vi "Part 2.vi"(11 "Input":string="on x=-44..5,y=-19..31,z=-15..33\non x=-39..11,y=-17..30,z=-15..30\non x=-42..10,y=-43..7,z=-4..40\non x=-4..47,y=-8..45,z=-8..43\non x=-18..28,y=-15..30,z=-36..12\non x=-24..24,y=-33..14,z=-49..1\non x=-14..30,y=-34..14,z=-27..24\non x=-45..7,y=-6..43,z=-9..41\non x=-16..37,y=-49..-5,z=-30..21\non x=-10..42,y=-35..10,z=-43..11\noff x=7..17,y=-8..5,z=-30..-18\non x=-49..3,y=-27..23,z=-44..1\noff x=10..23,y=-21..-10,z=-37..-19\non x=-41..4,y=-11..41,z=-36..16\noff x=-6..4,y=40..49,z=12..30\non x=-2..49,y=-43..3,z=-32..13\noff x=-44..-29,y=-8..6,z=1..17\non x=-9..36,y=-7..43,z=-37..14\noff x=-1..12,y=-36..-23,z=28..47\non x=-26..27,y=-45..3,z=-20..24\non x=-87853..-63955,y=-14079..10797,z=16618..34667\non x=-22600..-10441,y=-47268..-24491,z=-72641..-62383\non x=-7793..18488,y=71672..78114,z=-44666..-18458\non x=73..5701,y=-2494..28421,z=-89152..-65315\non x=-37051..-30202,y=15342..24015,z=-77231..-62996\non x=53246..70778,y=-62293..-47740,z=20277..41217\non x=-14142..12389,y=62146..65958,z=-55683..-41913\non x=-48728..-18398,y=8282..34289,z=-81114..-48336\non x=-59177..-22673,y=-49858..-29386,z=-59127..-47368\non x=-85434..-72245,y=13867..31427,z=-21594..-2631\non x=-35402..-12325,y=-37452..-19185,z=-81697..-63051\non x=61174..80227,y=-866..32461,z=-20053..-10077\non x=-32647..-1711,y=-35706..-20854,z=-72604..-60376\non x=59957..82200,y=-30164..2313,z=-30464..-19345\non x=6801..22281,y=24570..51370,z=-81154..-67264\non x=20369..39838,y=73729..88454,z=577..19763\non x=29800..52019,y=29499..61971,z=48435..55070\non x=28801..40411,y=-84420..-69983,z=-13267..2211\non x=13549..40576,y=-47493..-31658,z=-71685..-40487\non x=13137..24167,y=-66931..-49605,z=26517..54208\non x=33284..48135,y=46431..67202,z=48616..59067\non x=-56715..-26618,y=56864..79700,z=-25450..-654\non x=-54074..-25399,y=-52684..-36578,z=35631..52148\non x=37464..54023,y=-34067..-6521,z=-70559..-54490\non x=-41089..-11111,y=-47478..-29133,z=60940..74315\non x=-82774..-52991,y=-54204..-20897,z=23960..42825\non x=30749..49712,y=35786..69307,z=37491..45758\non x=-11491..14973,y=-93031..-58484,z=17353..44836\non x=-57064..-20188,y=-63440..-37103,z=47342..70176\non x=-27801..-375,y=30934..59690,z=45378..71236\non x=61123..82155,y=-15850..-525,z=-53874..-32638\non x=-16993..-2751,y=40182..64669,z=-62209..-45026\non x=-82058..-51602,y=6298..30885,z=-39693..-17573\non x=49260..58127,y=-59897..-48624,z=-30308..-16577\non x=-56788..-40095,y=-25293..-14542,z=-68269..-53982\non x=2505..5932,y=-47595..-22583,z=64838..84486\non x=-53828..-37906,y=-72105..-58994,z=-4913..17377\non x=5051..19306,y=77062..91570,z=-31347..-1735\non x=-16847..-320,y=-93124..-64459,z=12444..33910\non x=-45648..-18838,y=34175..55012,z=39079..55510\non x=63218..83253,y=-23970..-4735,z=2800..11596\non x=50244..76221,y=-50393..-33391,z=-17785..-7738\non x=35816..43139,y=-73177..-43183,z=-41697..-13098\non x=-66225..-48531,y=-36053..-16991,z=-48638..-26491\non x=-20786..8663,y=28061..38714,z=-84899..-63223\non x=59014..76501,y=10125..25324,z=-54183..-35850\non x=-24243..-8597,y=-47135..-12076,z=62724..76012\non x=-23347..7901,y=-81218..-55820,z=-60425..-30059\non x=56319..71652,y=23428..36372,z=-51760..-40670\non x=-13463..10312,y=78981..96298,z=-15494..17820\non x=25458..54307,y=-35736..-28250,z=48784..77696\non x=43259..63044,y=15682..26592,z=-71035..-52596\non x=-29348..-4953,y=54062..67679,z=39619..65019\non x=49369..63882,y=-39377..-21590,z=-53387..-47336\non x=13595..25896,y=27751..59875,z=-78381..-44266\non x=-62701..-44978,y=22333..30908,z=-54143..-42897\non x=7977..25840,y=-82123..-71218,z=-16092..-696\non x=72848..80580,y=-3963..7995,z=-14735..10441\non x=69499..92382,y=-2662..28065,z=-42992..-17994\non x=48475..68268,y=42740..64001,z=14503..39264\non x=-49063..-33385,y=-58610..-30409,z=41056..71840\non x=-59232..-33228,y=45184..76352,z=17766..31561\non x=5959..26638,y=-9552..20815,z=75305..87615\non x=47753..57971,y=42230..61946,z=-12647..-3804\non x=-81759..-73203,y=4440..38862,z=-16003..-3110\non x=-73980..-59456,y=-47097..-28017,z=-25117..7475\non x=23176..38914,y=50432..59832,z=31931..54668\non x=-71483..-48041,y=19572..30248,z=-40958..-32806\non x=-37783..-21743,y=-87276..-58240,z=-21390..-1919\non x=-18665..960,y=-5907..20986,z=66322..81301\non x=5286..37737,y=50107..67657,z=-67474..-42701\non x=31390..48914,y=-70366..-54470,z=-46904..-23117\non x=-27683..-15749,y=-47749..-34632,z=-76712..-50928\non x=-90781..-60103,y=-31150..-20145,z=-23382..5464\non x=-44373..-33411,y=55729..68596,z=-34550..-16532\non x=-1309..36490,y=-88067..-66282,z=-27329..-13890\non x=-70563..-54927,y=2742..28284,z=-59814..-41321\non x=36257..58977,y=52630..81787,z=-2016..28038\non x=59652..83384,y=-3386..9206,z=-40944..-13798\non x=-27792..6186,y=-47017..-27949,z=-75807..-45725\non x=60095..91023,y=-26573..-21046,z=-13267..10809\non x=-22369..-1689,y=-47418..-28289,z=-67790..-44667\non x=-73998..-62782,y=-24350..-3753,z=-44689..-24202\non x=-66355..-39116,y=26462..39518,z=44344..65908\non x=-82304..-51017,y=17614..36432,z=18664..50639\non x=-73956..-67827,y=18133..33852,z=-29108..-16920\non x=-79701..-67912,y=-30890..-20859,z=-11116..782\non x=60573..90823,y=-12009..12435,z=21040..48487\non x=-42470..-30925,y=18977..50582,z=-66812..-55290\non x=-44675..-19948,y=6997..36868,z=-76580..-55763\non x=-40167..-9959,y=-86179..-65330,z=22876..50418\non x=-14480..4184,y=-82281..-61373,z=-43344..-6589\non x=49703..56170,y=-12257..-3969,z=43782..66373\non x=37233..54010,y=-39264..-11480,z=-75787..-54270\non x=-63691..-41496,y=33366..47400,z=49232..66379\non x=-70135..-56354,y=-1294..17045,z=-54353..-30318\non x=-55679..-39187,y=-55170..-20576,z=-45155..-43051\non x=-68061..-60344,y=25128..55004,z=7484..41085\non x=39435..74411,y=-36766..-16956,z=-53809..-45526\non x=-17167..20391,y=13154..26529,z=75118..79685\non x=4750..24509,y=-2467..5837,z=-91364..-68976\non x=2296..23980,y=17845..29069,z=-78924..-67593\non x=-56852..-50617,y=9111..31762,z=40896..66920\non x=51868..71447,y=-10640..-4678,z=38788..67862\non x=37269..48010,y=-14504..-2446,z=51306..77677\non x=-78155..-61440,y=-2307..19061,z=-51692..-31851\non x=4082..21602,y=23861..44734,z=-72214..-55404\non x=-13005..1196,y=-94918..-62594,z=-26105..-7647\non x=12636..18371,y=-39962..-24982,z=71314..86048\non x=-59519..-38868,y=-32612..-26546,z=-52189..-29970\non x=50992..58060,y=1867..3995,z=-66397..-51090\non x=53023..64466,y=19765..49018,z=-47705..-32030\non x=54103..89259,y=32208..49754,z=18193..26605\non x=-54934..-44890,y=-32323..-24672,z=-57334..-43264\non x=21882..38565,y=-62552..-28774,z=37405..74274\non x=-14076..4166,y=-62802..-35587,z=-85575..-46763\non x=71563..94673,y=-28357..-5555,z=-8340..-3008\non x=-77691..-68006,y=16368..43879,z=6925..34881\non x=-62254..-44823,y=27169..57538,z=-43398..-29411\non x=-46115..-14147,y=23033..38605,z=-83660..-50766\non x=-81156..-69203,y=-2037..30876,z=-27757..-16747\non x=-64594..-49856,y=13230..41598,z=40946..48642\non x=74552..85238,y=-35069..-1080,z=-10139..5411\non x=48568..54268,y=15695..32917,z=-59194..-39272\non x=40963..56399,y=-43896..-32533,z=42647..66233\non x=-84712..-70637,y=-31823..-15214,z=5502..15753\non x=-50262..-43765,y=32260..44792,z=-56119..-43527\non x=-72959..-48790,y=-54165..-19818,z=21483..50707\non x=-75423..-57594,y=-44010..-34218,z=9567..42582\non x=46873..62215,y=-50840..-45150,z=3307..22080\non x=-51898..-33291,y=64961..76592,z=-1697..24644\non x=36342..50080,y=10355..34849,z=49771..76796\non x=-38727..-19183,y=22725..44395,z=56999..71498\non x=36920..68835,y=54496..74295,z=-578..22955\non x=-18190..-1806,y=79546..83150,z=-5596..16167\non x=-17085..4193,y=38116..44568,z=-83776..-59420\non x=60290..90016,y=-15660..4859,z=24..15702\non x=41898..73669,y=-29992..-11604,z=-69634..-37216\non x=22950..35763,y=39591..50067,z=-58475..-54162\non x=-83515..-76348,y=-24390..-7020,z=-5474..19494\non x=-12605..-6764,y=-9487..13991,z=-90796..-71648\non x=-84360..-56981,y=-6513..13663,z=10913..41809\non x=21065..50872,y=-77756..-54255,z=-32228..-10856\non x=-74731..-46649,y=-12397..8163,z=-61028..-48747\non x=-1567..17284,y=-29126..-8128,z=-83490..-65343\non x=23825..51820,y=-77978..-69264,z=-30297..474\non x=-2005..18443,y=-43669..-25998,z=-72518..-63834\non x=58982..72502,y=33029..35878,z=25466..40615\non x=51296..78353,y=24960..56356,z=-8313..18469\non x=-71399..-57843,y=-44261..-26742,z=22822..51410\non x=29760..36648,y=-4801..-3279,z=-85583..-66484\non x=40383..52091,y=42283..45005,z=-54444..-40795\non x=-28387..-13539,y=-5317..16212,z=-80930..-76037\non x=-42504..-32698,y=47026..63698,z=-43693..-30669\non x=-3125..32733,y=-61870..-39243,z=50456..68159\non x=9751..39005,y=10331..39830,z=64363..87555\non x=-86870..-68141,y=8031..39962,z=6587..42477\non x=-13099..12715,y=54037..72815,z=-53385..-32131\non x=14021..25542,y=42130..71403,z=40910..60362\non x=-6762..15002,y=-86093..-53378,z=31258..49920\non x=-17592..3127,y=-62373..-33600,z=53759..74959\non x=-89137..-56125,y=-35016..-8809,z=-30776..-5398\non x=44586..47260,y=22806..48955,z=-75476..-43472\non x=-40162..-24640,y=-57077..-35853,z=54246..71218\non x=-54201..-46541,y=-34915..-14935,z=52466..78173\non x=-6679..18857,y=45015..83502,z=-53804..-46675\non x=-62937..-53572,y=-35813..-29206,z=30508..53149\non x=-53689..-31763,y=-75022..-61400,z=-12035..7506\non x=-24770..-7480,y=-70530..-33052,z=47004..67401\non x=-64788..-42202,y=-34456..-14089,z=-58243..-36384\non x=-41276..-16521,y=-57613..-37888,z=-69142..-40440\non x=-25613..-2328,y=48311..67290,z=44223..57924\non x=-90192..-58384,y=-12961..-7477,z=5935..23214\non x=16121..48809,y=-60926..-51273,z=-43839..-30861\non x=26638..60652,y=-44537..-30587,z=58405..71906\non x=-66410..-36432,y=42454..70443,z=-23159..-10037\non x=-71864..-54435,y=-36243..-23995,z=14596..34041\non x=9052..28723,y=-77203..-70603,z=-31838..-18146\non x=-4816..25036,y=61688..76240,z=21251..46199\non x=61863..71834,y=-7068..7469,z=29122..46978\non x=-53069..-22747,y=-61003..-50886,z=-41977..-36808\non x=-66306..-36754,y=-45013..-22032,z=-44535..-24946\non x=62478..87269,y=10773..28720,z=22334..42400\non x=14448..43447,y=-90837..-63542,z=-24857..-11445\non x=-6219..24505,y=2176..20741,z=65816..91491\non x=-4504..16125,y=26649..38859,z=-75806..-66094\non x=-7593..12762,y=10851..31680,z=75476..87589\non x=-77806..-73411,y=-6826..6277,z=-35741..-6990\non x=-16506..5646,y=-39393..-25156,z=-93753..-55332\non x=-32247..1348,y=72630..91477,z=15827..32435\non x=-19625..-6807,y=-67138..-42260,z=-72627..-49737\non x=-53034..-25232,y=-36424..-7517,z=-81260..-66867\non x=9597..27791,y=-44126..-18665,z=-77320..-64055\non x=36930..61974,y=-53931..-23875,z=-56634..-50103\non x=-80031..-64462,y=29885..46965,z=-25547..-6196\non x=-66414..-43495,y=36573..62850,z=-24776..-6505\non x=-25011..-9028,y=-69426..-56148,z=40533..73395\non x=25534..46636,y=46058..52691,z=45249..72792\non x=-7618..10902,y=17884..23097,z=66984..80601\non x=-83176..-71251,y=-32175..-7710,z=-922..21556\non x=29449..65515,y=-51110..-34476,z=34096..63188\non x=-3631..24310,y=-20299..-15069,z=72984..92165\noff x=-50424..-41375,y=-72654..-44771,z=838..16943\non x=3025..40907,y=-78511..-53856,z=42248..53660\noff x=-29442..-18169,y=33929..64130,z=58394..78342\non x=62016..93099,y=-36239..-22606,z=-10475..12016\noff x=-81393..-49724,y=10305..34270,z=34305..51924\noff x=31937..42583,y=14977..40524,z=55574..83356\noff x=-72488..-54163,y=21000..44643,z=-45612..-27454\noff x=-93753..-69438,y=3271..31377,z=-16945..2818\noff x=13847..37017,y=35958..73486,z=47726..60893\non x=-75263..-59456,y=36203..54394,z=-2931..20048\noff x=27162..44008,y=-59493..-34872,z=51686..75220\noff x=-73602..-38606,y=35904..52123,z=-42290..-18989\noff x=-73300..-45099,y=-10701..14399,z=-59463..-39706\noff x=-83528..-62414,y=1442..31990,z=39787..61495\non x=-19227..1177,y=-81493..-56654,z=33563..39495\noff x=-70257..-52022,y=-44692..-24441,z=-30358..1873\noff x=-94684..-63304,y=-18953..-12160,z=-1247..15579\non x=4516..21971,y=-26822..-8920,z=-92246..-59738\non x=47592..59821,y=28110..44046,z=27804..52573\non x=39539..58512,y=41354..52402,z=33137..45594\non x=41004..62753,y=-62983..-58912,z=233..14053\non x=43897..71120,y=2903..24584,z=47215..77087\non x=-62187..-30271,y=-53081..-44707,z=-46266..-28266\noff x=46434..73444,y=-53205..-35815,z=-57794..-35076\non x=-87521..-71461,y=-28669..-7399,z=-4329..4473\noff x=14524..33155,y=-74653..-59465,z=7788..40782\noff x=42666..81619,y=17492..36905,z=38287..62402\non x=-8726..16759,y=-24348..-2024,z=-90211..-65111\non x=49994..62962,y=2227..24922,z=41992..62455\non x=30619..39110,y=44325..68006,z=29475..58157\non x=52166..86859,y=-16051..-2288,z=-35893..-16028\noff x=-82950..-67164,y=-38616..-23530,z=2815..26199\noff x=15592..49678,y=-59501..-50916,z=-71638..-51719\non x=-5599..2448,y=-4875..22375,z=63268..95230\noff x=-26144..-7146,y=30378..40422,z=54534..80457\noff x=-67364..-46592,y=-8423..11830,z=-62371..-57595\noff x=19562..40225,y=35029..49193,z=-72197..-56945\noff x=-64792..-35048,y=28984..33453,z=-64967..-42923\non x=2826..26378,y=-85400..-49030,z=22072..48794\non x=-3048..15987,y=23466..47779,z=60807..88012\noff x=-43613..-23923,y=-21725..13753,z=-74679..-71666\non x=57515..73257,y=4463..19735,z=-55663..-40576\noff x=-71509..-36371,y=-44288..-32500,z=-58805..-43879\noff x=4058..10573,y=-90040..-74031,z=-11420..15283\non x=11578..34158,y=43086..64864,z=48987..55683\noff x=-90937..-61197,y=-42619..-7059,z=-13526..6975\non x=-47775..-35341,y=21796..40791,z=-74978..-54225\non x=55459..86075,y=-33737..-10240,z=-38803..-31160\non x=66900..95307,y=-658..33987,z=2578..31976\non x=51781..62459,y=11954..37284,z=-55567..-29845\non x=7564..38303,y=24656..45979,z=58307..72979\noff x=25925..40008,y=7133..29683,z=66022..81463\noff x=16087..31819,y=-49297..-18917,z=49254..81722\non x=61816..77023,y=32302..50207,z=-26122..-13342\non x=-16944..-551,y=27348..36381,z=51222..84114\non x=-60896..-35718,y=-25770..-3198,z=-73389..-51938\non x=53570..57442,y=-56748..-34158,z=28231..37748\noff x=12948..34050,y=-89722..-76481,z=5288..20288\non x=4092..16941,y=33046..61784,z=62511..75003\non x=-34294..-19056,y=40621..66504,z=50350..66716\noff x=-60552..-37543,y=25044..37455,z=-67217..-44428\non x=-59672..-43404,y=-44998..-33041,z=24549..48963\noff x=11363..42189,y=-34219..-11130,z=65796..73487\non x=-5878..3795,y=-82227..-65797,z=-55000..-37476\noff x=-44704..-16546,y=-53365..-29060,z=63096..82254\noff x=46835..59255,y=42974..52180,z=38447..52668\non x=28649..53034,y=69128..86256,z=-27036..-4069\non x=31797..51935,y=-70873..-40006,z=27113..55156\non x=-16413..784,y=74995..86748,z=22251..36557\noff x=-51126..-19696,y=62556..79243,z=13535..24185\non x=55195..69351,y=16387..17587,z=-68210..-51399\noff x=-12380..3805,y=-37523..-6086,z=-84246..-72810\non x=-7904..10345,y=-43424..-9185,z=-81538..-63642\non x=9595..28061,y=-57291..-53511,z=41104..58415\non x=-22057..-8429,y=-74023..-50595,z=-53834..-25785\noff x=39543..72810,y=43357..57907,z=-4967..5825\non x=25952..46891,y=-59512..-39577,z=-66604..-42237\noff x=-45845..-9503,y=21188..47233,z=-73595..-46458\noff x=-58705..-40574,y=40410..62602,z=37852..56809\noff x=42166..60256,y=15546..23665,z=-62954..-50742\non x=-54920..-38787,y=-73440..-55858,z=-22924..-10148\non x=-21604..70,y=-67168..-37800,z=-73842..-58943\non x=44585..52863,y=-47677..-38099,z=32512..59378\noff x=-68847..-37762,y=-79749..-45298,z=-31814..-6826\non x=65721..82686,y=32570..53560,z=-35607..-1198\non x=-78244..-53156,y=5914..35587,z=34459..50180\non x=-88381..-63342,y=13742..41912,z=-47591..-12686\noff x=39744..59977,y=38226..43544,z=34889..57448\noff x=67454..97825,y=-3852..18383,z=-27139..2873\non x=-52994..-36607,y=-3822..8882,z=42832..75144\noff x=29703..50057,y=6444..44725,z=60091..61494\noff x=49384..69382,y=23037..31241,z=30044..58530\non x=77544..93200,y=-18366..4222,z=-12443..9543\non x=32444..48168,y=-80604..-46813,z=23017..35539\non x=-54080..-41598,y=-75034..-61527,z=17545..24716\non x=-41183..-15966,y=57318..88966,z=-13329..645\noff x=47462..69587,y=41234..55751,z=7512..26329\noff x=20009..45002,y=4144..8442,z=-86914..-66660\noff x=-73916..-62216,y=5685..32016,z=12725..39661\non x=-14035..-6506,y=-83445..-75166,z=-1527..27655\non x=-30238..-19986,y=-24777..-2077,z=-77292..-64543\non x=64167..87115,y=-14177..14758,z=-10742..8450\non x=25780..55516,y=-55330..-54111,z=-49841..-36268\non x=-52479..-29315,y=20462..47890,z=-73960..-60169\noff x=-76016..-57381,y=19112..40178,z=548..19861\noff x=-8311..28174,y=35103..47065,z=55844..85226\non x=47293..59980,y=-45343..-28831,z=-44151..-25784\noff x=519..30306,y=62364..90147,z=-39751..-13511\non x=-80316..-68742,y=708..27017,z=3955..23948\noff x=-70769..-49823,y=38737..57694,z=-7758..18891\non x=48446..72061,y=33800..62229,z=13535..45267\non x=-16168..2997,y=-22975..-8077,z=66199..85132\non x=-64980..-35565,y=-66241..-53278,z=-7348..-3672\non x=-91717..-65980,y=-44249..-12365,z=-10984..8372\noff x=35322..39858,y=-27123..-8496,z=-77757..-48994\non x=-3930..26786,y=7461..23065,z=72518..91768\noff x=-10532..-7074,y=-11464..-3902,z=-89986..-72527\non x=53629..81615,y=-60075..-45846,z=-12320..14928\noff x=-83656..-68996,y=-18080..13189,z=-29337..-11467\non x=-46774..-28700,y=-23827..-6270,z=54246..76853\non x=-41689..-29588,y=-38149..-13551,z=64995..75004\non x=15365..46478,y=-84175..-57499,z=-26982..-18015\non x=8773..29446,y=4874..31204,z=-76125..-63650\noff x=60322..94998,y=-27912..-3665,z=11178..26231\non x=19730..29512,y=64835..89598,z=-15849..-1111\noff x=63457..87596,y=-8272..9336,z=-8510..14156\non x=36965..68511,y=-65996..-38254,z=-37353..-20861\noff x=2138..11555,y=5930..21645,z=76602..92006\noff x=69350..83044,y=-1970..18069,z=-34741..-436\non x=-25153..-8758,y=-26143..-17681,z=67900..79657\noff x=53321..63311,y=55770..63844,z=-6768..8042\noff x=51015..78137,y=-33031..-8895,z=-61391..-32324\non x=-79490..-58269,y=31453..57687,z=-11468..21464\non x=-3275..13773,y=-60815..-44132,z=-65158..-49441\non x=-68779..-46445,y=34511..50996,z=11030..50059\noff x=-8177..9317,y=-24563..-19731,z=-90510..-57472\noff x=48390..66333,y=9511..33396,z=-64098..-38743\non x=26868..41962,y=-25709..-9549,z=-81852..-64083\noff x=40254..56776,y=3315..23418,z=44927..57319\noff x=-38532..-18812,y=-34537..-3999,z=67871..72424\non x=-80451..-54109,y=8141..28630,z=40649..48488\noff x=-41866..-33082,y=48481..67972,z=34669..38558\non x=1985..11485,y=-5625..16920,z=-83211..-61053\non x=-50296..-25997,y=-50861..-39499,z=-65512..-50437\non x=-76530..-46217,y=36628..58187,z=14709..31320\noff x=-36064..-11086,y=61197..84224,z=-23954..8344\non x=-20066..-13478,y=62687..90046,z=-44287..-15529\non x=-37373..-11863,y=-76819..-55289,z=12018..28023\noff x=54893..70941,y=6313..31555,z=42682..63276\noff x=71444..90185,y=-19742..-5636,z=-48222..-17689\noff x=-14573..7088,y=73450..80278,z=-26894..-20381\non x=-63000..-52387,y=33041..69197,z=-25867..-1432\noff x=-27022..-20859,y=69040..75320,z=-17231..5175\non x=-19675..-10057,y=6582..22912,z=-94740..-73605\non x=-60861..-29005,y=-54918..-22947,z=47523..63863\non x=39472..51894,y=45318..61684,z=6788..38771\noff x=-55953..-40048,y=-59964..-45678,z=17400..37433\noff x=-73856..-61903,y=29214..41492,z=-4021..14451\non x=-5749..21764,y=70076..88432,z=15120..37797\noff x=-77673..-56604,y=-68356..-48827,z=-15377..-3043\noff x=50082..86960,y=10169..33250,z=-44586..-26970\noff x=44499..52189,y=-19697..-760,z=52574..68835\non x=10922..32585,y=-72130..-55088,z=-44965..-19204\noff x=-9238..16630,y=57174..87938,z=-50830..-23199\noff x=19787..51570,y=30181..54089,z=53955..68032\non x=-85972..-64552,y=-26460..-7515,z=-2073..20090\non x=2449..30075,y=50071..72688,z=-46982..-43059\noff x=-52224..-35101,y=12040..27039,z=57095..68801\non x=-52590..-20949,y=63328..67968,z=20767..40966\noff x=-7170..16103,y=-45147..-39116,z=54536..68891\non x=-43865..-21841,y=16142..32004,z=-79917..-62289\non x=-33415..-17146,y=11743..48210,z=52933..77317\noff x=26648..53644,y=9918..29253,z=-84770..-63255\noff x=-25080..-17950,y=-46679..-19928,z=60760..87410\non x=28049..53541,y=32306..58979,z=32761..48445\non x=-15099..19253,y=-51961..-27400,z=-78713..-62878\noff x=5435..29239,y=-82008..-74434,z=-25893..-5850\non x=-84963..-58158,y=31674..43258,z=-20003..886\noff x=-56694..-44118,y=22049..31804,z=48676..56434\non x=59174..61663,y=-61770..-27812,z=10113..42440\noff x=34585..61402,y=34615..61628,z=-34172..-13772\noff x=-81862..-53602,y=45469..58334,z=-25538..1498\non x=-34692..-20244,y=-35779..-11661,z=-78349..-57042\non x=-67354..-46237,y=15178..48955,z=-64336..-47149\noff x=9659..35954,y=-14803..1942,z=-92105..-70797\non x=-50655..-24121,y=52828..57401,z=40182..48460\noff x=51557..75536,y=-50906..-42455,z=-1724..17091\noff x=-21560..5780,y=56640..95726,z=10768..39375\noff x=6098..35818,y=-68926..-41836,z=38622..61618\non x=-11245..8010,y=54297..85302,z=18748..48445\non x=48474..77047,y=17887..37948,z=33470..46973\noff x=66358..89307,y=-141..8414,z=-46824..-19030\non x=-516..19961,y=60846..83692,z=7191..24993\noff x=-40080..-11830,y=-6526..24432,z=56923..92614\non x=-71762..-54288,y=-30785..-3150,z=29701..47370\noff x=-82694..-66540,y=-33056..-10908,z=-42820..-19656\non x=27229..53914,y=44050..57314,z=44689..70835\non x=4204..33386,y=59417..88203,z=18434..23931") -> (3 "Output":i64=1217808640648260)   [LabVIEW 2021]
uses:
  9a6a6488-fe01-433a-8c08-ec40a0e1c2a6.vi
panel:
  out "size(s)":i32=48752
  out "Progress":dbl=100.0
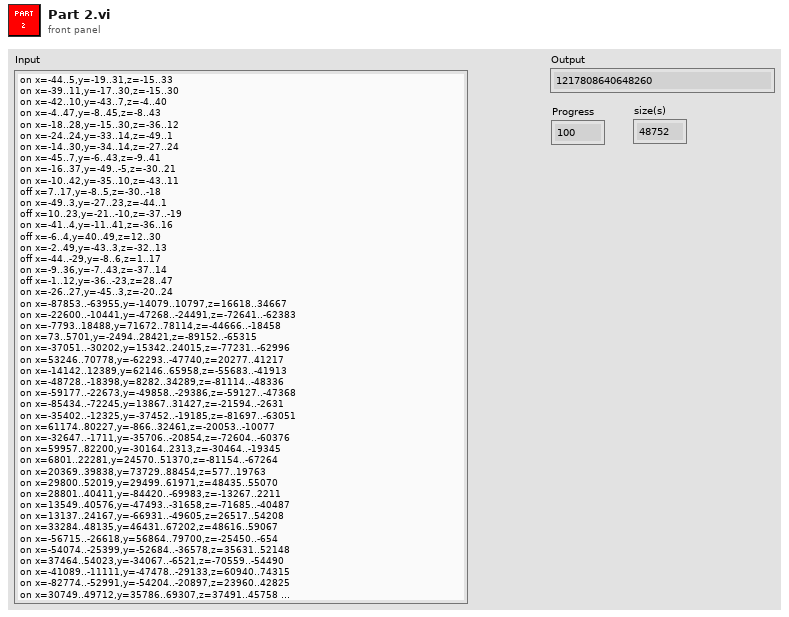
[diagram p1: front panel]
types:
  T1 = cluster{"X Min":i64, "X Max":i64, "Y Min":i64, "Y Max":i64, "Z Min":i64, "Z Max":i64}
  T2 = cluster{"X Min":i64, "X Max":i64, "Y Min":i64, "Y Max":i64, "Z Min":i64, "Z Max":i64}[]
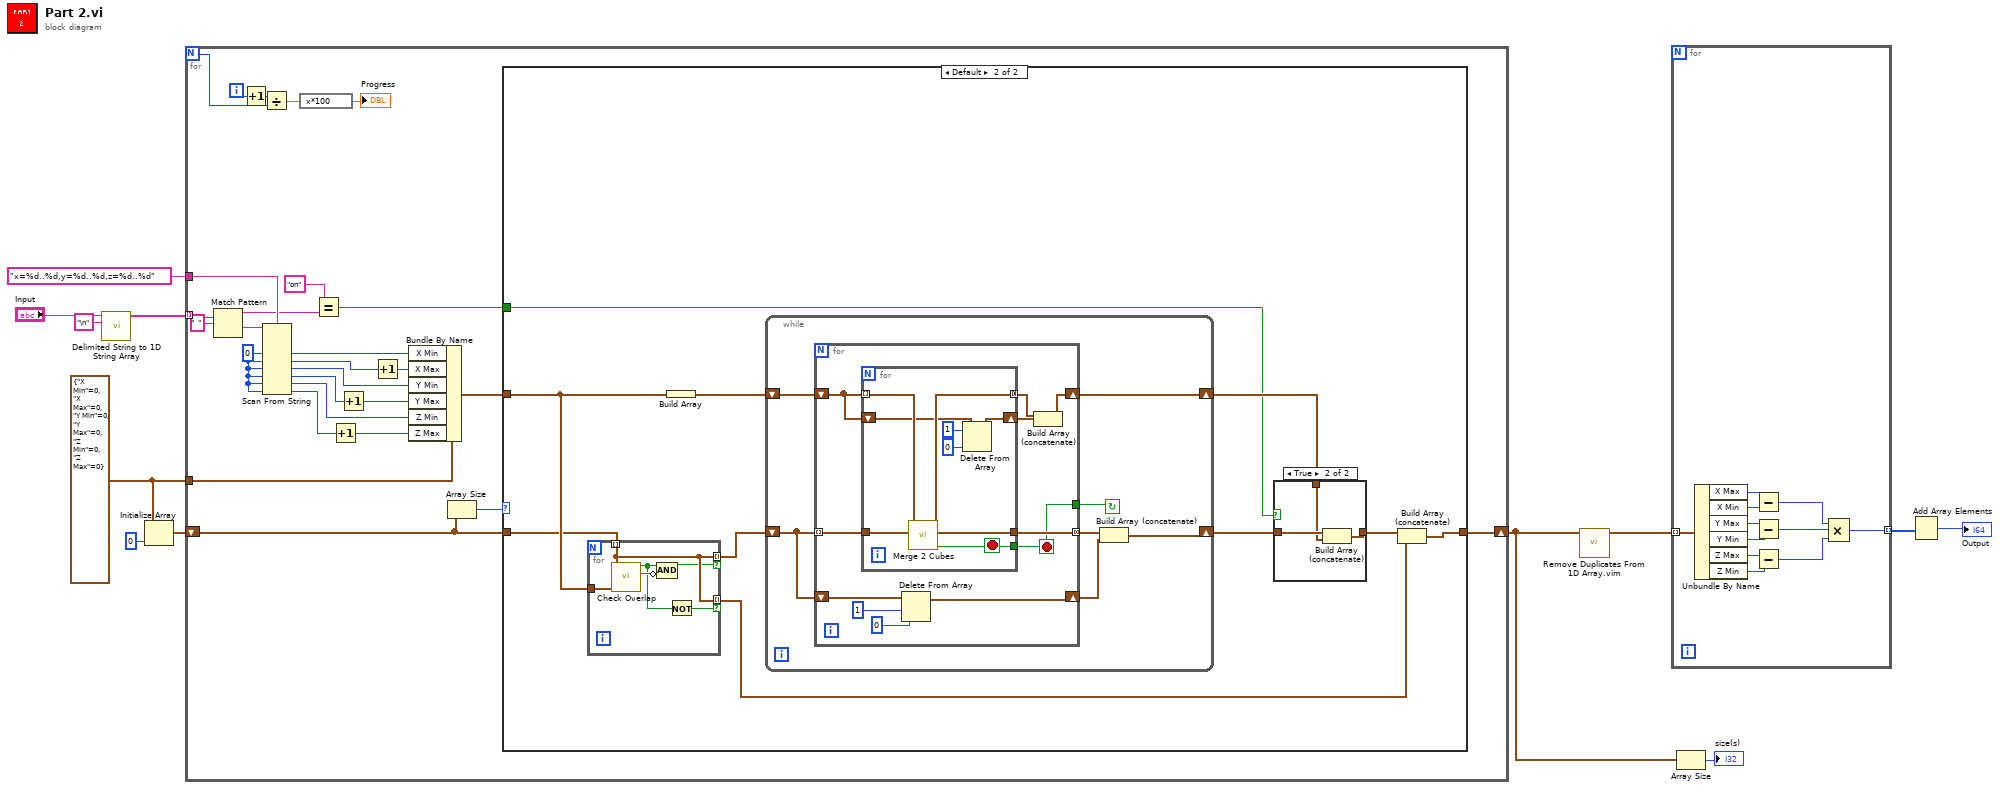
[diagram p0: block diagram]
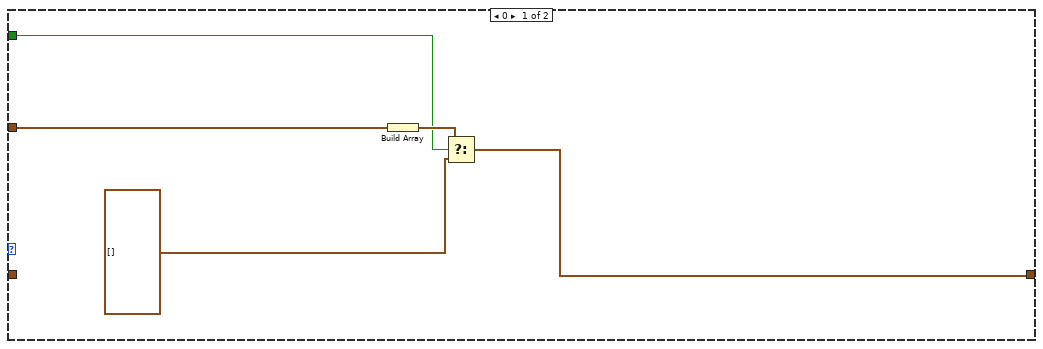
[diagram p2: hidden frame]
diagram:
  w7 = T1 {"X Min"=0, "X Max"=0, "Y Min"=0, "Y Max"=0, "Z Min"=0, "Z Max"=0}
  n1 = call <vilib>:"Delimited String to 1D String Array.vi"("delimiter"="\n", "delimited string"="Input") -> ("string array"=w3:string[])  [unwired: 9 in]
  n2 = Initialize Array(w7, 0 ("dimension size")) -> (w9:T2)
  n3 = for {
    N -> [w31]
    tunnel: w3 -> [w39] mode=indexing
    tunnel: "x=%d..%d,y=%d..%d,z=%d..%d" ("format string") -> [w37]
    tunnel: w7 -> [w27]
    shift-right: [w18] -> w4
    shift-left: w9 -> [w20]
    i -> [w32]
    w34 = i64 0 ("default value 1")
    n4 = Match Pattern(string=w39, regular expression=" ") -> (before substring=w36:string, after substring=w38:string)  [unwired: 1 in, 2 out]
    n5 = Increment(x=w32) -> (x+1=w17:i32)
    n6 = Divide(x=w17, y=w31) -> (x/y=w30:dbl)
    n7 = Scan From String(format string=w37, input string=w38, default 1=w34, default 2=w34, default 3=w34, default 4=w34, default 5=w34, default 6=w34) -> (output 1=w28:i64, output 2=w13:i64, output 3=w26:i64, output 4=w25:i64, output 5=w24:i64, output 6=w23:i64)  [unwired: 2 in, 3 out]
    n8 = expression code="x*100"(w30) -> (→"Progress":dbl)
    n9 = Equal?(x="on", y=w36) -> (x = y?=w21:bool)
    n10 = Increment(x=w23) -> (x+1=w15:i64)
    n11 = Increment(x=w25) -> (x+1=w16:i64)
    n12 = Increment(x=w13) -> (x+1=w14:i64)
    n13 = Bundle By Name(cluster=w27, "X Min"=w28, "X Max"=w14, "Y Min"=w26, "Y Max"=w16, "Z Min"=w24, "Z Max"=w15) -> (w22:T1)
    n14 = Array Size(array=w20) -> (size(s)=w19:i32)
    n15 = case shown="Default" w19 {
      tunnel: w22 -> [w44 w49]
      tunnel: w21 -> [w40 w52]
      tunnel: [w41 w46] -> w18
      tunnel: w20 -> [_ w48]
      frame 0 {
        n16 = Build Array(w44) -> (w42:T2)
        n17 = Select(t=w42, s=w40, f=T2 [] ("On Cubes")) -> (s? t:f=w41:T2)
      }
      frame Default {
        n18 = for {
          tunnel: w49 -> [w60]
          tunnel: w48 -> [w59] mode=indexing
          tunnel: [w59] -> w47 mode=indexing if=w57
          tunnel: [w59] -> w45 mode=indexing if=w55
          n19 = call "Check Overlap.vi"("Cube 2"=w60, "Cube 1"=w59) -> ("Full Overlap?"=w58:bool, "Overlap?"=w56:bool)  [unwired: 8 in]
          n20 = Compound Arithmetic op=AND(w56, invert w58) -> (w57:bool)
          n21 = Not(x=w56) -> (.not. x?=w55:bool)
        }
        n22 = Build Array(w49) -> (w54:T2)
        n23 = while {
          shift-right: [w65] -> w53
          shift-left: w54 -> [w66]
          shift-right: [w67] -> w51
          shift-left: w47 -> [w64]
          stop <- w61 continue-if-true
          n24 = for {
            tunnel: w64 -> [w78] mode=indexing
            tunnel: [w77] -> w62 mode=concatenating
            shift-right: [w73] -> w65
            shift-left: w66 -> [w74]
            shift-right: [w75] -> w63
            shift-left: w64 -> [w76]
            tunnel: [w72] -> w61
            stop <- w72 stop-if-true
            n25 = for {
              tunnel: w78 -> [w87]
              tunnel: [w86] -> w77
              tunnel: w74 -> [w85] mode=indexing
              tunnel: [w84] -> w68 mode=concatenating
              shift-right: [w80] -> w69
              shift-left: w74 -> [w81]
              tunnel: [w79] -> w72
              stop <- w79 stop-if-true
              n26 = call "Merge 2 Cubes.vi"("Cube 1"=w87, "Cube 2"=w85) -> ("Overlap?"=w79:bool, "Cube 1 Parts"=w86:T2, "Cube 2 Parts"=w84:T2)  [unwired: 7 in]
              n27 = Delete From Array(array=w81, length=1, index=0) -> (array with subset deleted=w80:T2)  [unwired: 1 out]
            }
            n28 = Delete From Array(array=w76, length=1, index=0) -> (array with subset deleted=w75:T2)  [unwired: 1 out]
            n29 = Build Array (concatenate)(w68, w69) -> (w73:T2)
          }
          n30 = Build Array (concatenate)(w62, w63) -> (w67:T2)
        }
        n31 = case shown="True" w52 {
          tunnel: w51 -> [w88 w91]
          tunnel: [w88 w90] -> w50
          tunnel: w53 -> [_ w89]
          frame False {
          }
          frame True {
            n32 = Build Array (concatenate)(w91, w89) -> (w90:T2)
          }
        }
        n33 = Build Array (concatenate)(w50, w45) -> (w46:T2)
      }
    }
  }
  n34 = call "Remove Duplicates From 1D Array.vim"("array"=w4) -> ("array with duplicates removed"=w1:T2)  [unwired: 10 in]
  n35 = for {
    tunnel: w1 -> [w102] mode=indexing
    tunnel: [w92] -> w2 mode=indexing
    n36 = Unbundle By Name(w102) -> ("X Max"=w96:i64, "X Min"=w97:i64, "Y Max"=w98:i64, "Y Min"=w99:i64, "Z Max"=w101:i64, "Z Min"=w100:i64)
    n37 = Subtract(x=w96, y=w97) -> (x-y=w93:i64)
    n38 = Subtract(x=w98, y=w99) -> (x-y=w95:i64)
    n39 = Subtract(x=w101, y=w100) -> (x-y=w94:i64)
    n40 = Compound Arithmetic op=MULTIPLY(w93, w95, w94) -> (w92:i64)
  }
  n41 = Array Size(array=w4) -> (size(s)=→"size(s)":i32)
  n42 = Add Array Elements(numeric array=w2) -> (sum=→"Output":i64)
